vi "Type.vi"(11 "IntegerPanel in":refnum<class "IntegerPanel.lvclass">) -> (2 "Type":refnum<class "Type.lvclass">)   [LabVIEW 2020, in "Conditum-Tools.lvlib" / "IntegerPanel.lvclass"]
uses:
  IntegerPanel.lvclass
  Conditum/Columns/Type/Type.lvclass
  IntegerPanel.lvclass/IntegerPanel.ctl
  Conditum/Columns/Integer/Integer.lvclass
  C:/dev/lv20CE/lv-conditum/Conditum/Columns/Type/Type.lvclass
  C:/dev/lv20CE/lv-conditum/Conditum/Columns/Integer/Integer.lvclass
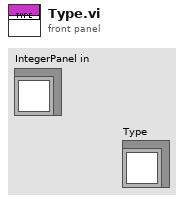
[diagram p1: front panel]
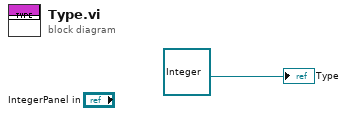
[diagram p0: block diagram]
diagram:
  "Type" <- refnum<class "Integer.lvclass"> refnum ("Conditum:Columns:Integer.lvclass")
